vi "medicion_digital_task.vi"() -> ()   [LabVIEW 2024]
uses:
  <vilib>/DAQmx/read.llb/DAQmx Read (Digital 1D Bool NChan 1Samp 1Line).vi
  <vilib>/DAQmx/miscellaneous.llb/DAQmx Fill In Error Info.vi
panel:
  in  "stop":bool
  out "data":bool[](array[boolean])
  in  "task/channels in":refnum<k21>
  # "Se leen las entradas digitales utilizando una \"task\"\nconfigurada en NI MAX con el nombre \"read_collector\""
  # "DAQ utilizado NI USB 6009"
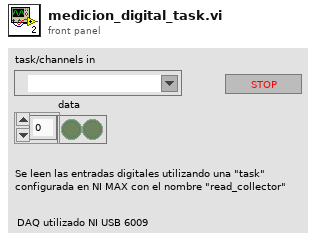
[diagram p1: front panel]
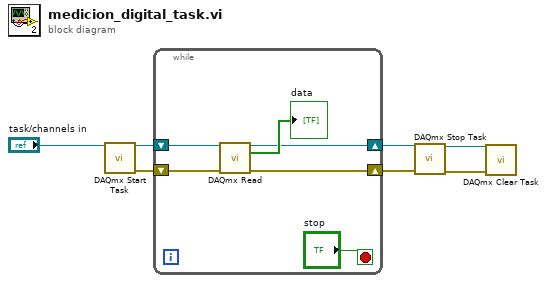
[diagram p0: block diagram]
diagram:
  n1 = call <vilib>:"DAQmx Start Task.vi"("task/channels in"="task/channels in") -> ("task out"=w7:refnum<k21>, "error out"=w6:errorcluster)  [unwired: 13 in]
  n2 = while {
    shift-right: [w10] -> w4
    shift-left: w7 -> [w13]
    shift-right: [w9] -> w3
    shift-left: w6 -> [w12]
    stop <- "stop" stop-if-true
    n3 = call-poly <vilib>:"DAQmx Read.vi"("task/channels in"=w13, "error in"=w12) -> ("task out"=w10:refnum<k21>, "data"=→"data":bool[], "error out"=w9:errorcluster)  [unwired: 11 in]
  }
  n4 = call <vilib>:"DAQmx Stop Task.vi"("task/channels in"=w4, "error in"=w3) -> ("task out"=w2:refnum<k21>, "error out"=w1:errorcluster)  [unwired: 12 in]
  n5 = call <vilib>:"DAQmx Clear Task.vi"("task in"=w2, "error in"=w1) -> ()  [unwired: 13 in, 1 out]
